vi "VI Messdaten-Verteiler.vi"(8 "error in (no error)":errorcluster caption="Fehler (Eingang, kein Fehler)") -> (0 "error out":errorcluster caption="Fehler (Ausgang)")   [LabVIEW 2020, in "Messdaten.lvlib"]
uses:
  Messdaten/Messdaten.lvlib
  Messdaten/Aktionen FGV Messdaten logging.ctl
  Seiten/Log Konfig/Aktionen Logdatei erstellen.ctl
  Seiten/FT-IR/FGV FT-IR Aktionen.ctl
  Allgemein/Zykluszeiterfassung Aktionen.ctl
  Seiten/System Einstellungen V2/Aktioen FGV System.ctl
  Messdaten/Aktionen FGV Messwerte zusammenfassen.ctl
  Seiten/FT-IR/FGV FT-IR Diagnose Aktionen.ctl
  Seiten/FT-IR/FGV FT-IR Gasliste Aktionen.ctl
  Status Analysatoren/Aktion Status Analysatoren.ctl
  Seiten/Log Konfig/Aktionen LogFile schreiben.ctl
  Seiten/Log Konfig/Aktionen Trigger.ctl
  Seiten/EL3000/Allgemeine VI/Aktion FGV Werte Standardanalysator.ctl
  Seiten/FT-IR/Algebraic Modul/FGV Algebraic Aktionen.ctl
  Seiten/FT-IR/Aktionen EVID-Codes.ctl
  Messdaten/Aktionen FGV Messdaten.ctl
  Seiten/Log Konfig/Log Sequence FGV Aktion.ctl
  Seiten/FT-IR/FT-IR.lvlib
  Seiten/FT-IR/TOOLweb Interface Library/TOOLweb Interface.lvlib
  cRIO/PC/Kommunikation mit cRIO.lvlib
  Seiten/Log Konfig/LogKonfig.lvlib
  Seiten/FT-IR/AK interface/AK-Interface.lvlib
  Allgemein/allgemeine Sub-VIs.lvlib
  Seiten/EL3000/PMA/PMA.lvlib
  Seiten/EL3000/FID/FID.lvlib
  Seiten/EL3000/Allgemeine VI/Allgemeine VI.lvlib
  Seiten/FT-IR/Algebraic Modul/Algebraic Modul.lvlib
  Seiten/Lambdasonde/Lambda_ Komm.lvlib
  Status Analysatoren/Status Analysatoren.lvlib
  Linearisierung V2/Linearisierung v2.lvlib
  <vilib>/Platform/TimedLoop/XDataNode/XDataNode.xnode
  <vilib>/Platform/TimedLoop/XDataNode/nitl_modes.ctl
  <vilib>/Platform/TimedLoop/XDataNode/XDNodeRunTimeDep.lvlib
  <vilib>/Platform/TimedLoop/XDataNode/wakeup.ctl
  <vilib>/Platform/TimedLoop/XDataNode/timing_clust.ctl
  Seiten/FT-IR/TOOLweb Interface Library/TOOLweb Interface Hilfs-VIs.lvlib
  Seiten/System Einstellungen V2/System Einstellungen V2.lvlib
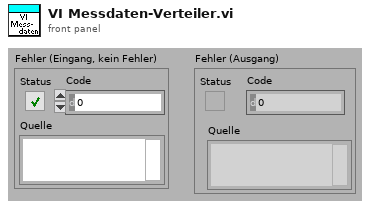
[diagram p1: front panel]
types:
  T1 = typedef "Messdaten.lvlib/Aktionen FGV Messdaten logging.ctl" = enum16{"lesen", "schreiben", "init", "löschen", "werte eintakten", "Flag setzen"}
  T2 = typedef "XDNodeRunTimeDep.lvlib/timing_clust.ctl" = cluster{"Expected End [f-1]":u64, "Actual End [f-1]":u64, "Finished Late? [f-1]":bool, "Expected End [i-1]":u64, "Actual End [i-1]":u64, "Finished Late? [i-1]":bool, "Expected Start [i]":u64, "Actual Start [i]":u64, "Expected Start [f]":u64, "Actual Start [f]":u64, "Source Name":string, "Structure Name":string, "Period":i64, "Deadline":i64, "Offset":i64, "Start":i64, "Priority":i32, "Timeout":i32, "Mode":T3, "Wakeup Reason":T4, "Error":errorcluster, "Source Type":string, "Secondary Source Type":string, "Global End Time":u64, "Global Start Time":u64, "Frame Duration":u64, "Iteration Duration":u64, "Assigned CPU":i32, "I/O Scan Engine Mode":u32}
  T3 = typedef "XDNodeRunTimeDep.lvlib/nitl_modes.ctl" = enum32{"No Change", "Process missed periods, maintain original phase", "Discard missed periods, maintain original phase", "Process missed periods, ignore original phase", "Discard missed periods, ignore original phase"}
  T4 = typedef "XDNodeRunTimeDep.lvlib/wakeup.ctl" = enum32{"Normal", "Aborted", "Asynchronous wakeup", "Timing source error", "Timed loop error", "Timeout"}
  T5 = typedef "System Einstellungen V2.lvlib/Aktioen FGV System.ctl" = enum16{"lesen", "laden", "speichern", "Optionen schreiben", "Zeitstempel", "Reset BMP", "Reset SQP", "Wartung", "Werkseinstellung"}
  T6 = typedef "allgemeine Sub-VIs.lvlib/Zykluszeiterfassung Aktionen.ctl" = enum16{"lesen", "init", "Messdaten1", "ToolWeb", "AK FT-IR", "AK Extern", "AK Amium"}
  T7 = typedef "FT-IR.lvlib/FGV FT-IR Aktionen.ctl" = enum16{"lesen", "NOG setzen", "NOS setzen", "Initialisieren", "speichern", "ALLES setzen", "FT-IR Spektrum loggen", "Komm Stoppen", "Spektrum LogKonfig"}
  T8 = typedef "Messdaten.lvlib/Aktionen FGV Messdaten.ctl" = enum16{"lesen", "schreiben", "löschen", "Mittelwerte", "Komponente"}
  T9 = typedef "FT-IR.lvlib/Aktionen EVID-Codes.ctl" = enum16{"lesen", "setzen", "laden", "speichern", "1Hz/5Hz", "Smoothing", "Rolling Average"}
  T10 = typedef "FT-IR.lvlib/Algebraic Modul.lvlib/FGV Algebraic Aktionen.ctl" = enum16{"lesen", "laden", "speichern", "berechnen", "schreiben"}
  T11 = typedef "ABB-EL3000.lvlib/Allgemeine VI.lvlib/Aktion FGV Werte Standardanalysator.ctl" = enum16{"lesen", "FID", "PMA"}
  T12 = typedef "Messdaten.lvlib/Aktionen FGV Messwerte zusammenfassen.ctl" = enum16{"lesen", "FT-IR", "Algebraic", "LabBaseName", "LabBaseNr"}
  T13 = typedef "LogKonfig.lvlib/Aktionen Trigger.ctl" = enum16{"lesen", "ALLE schreiben", "Trigger prüfen", "Trigger rücksetzen"}
  T14 = typedef "LogKonfig.lvlib/Log Sequence FGV Aktion.ctl" = enum16{"initialisieren", "lesen", "schreiben", "laden", "speichern", "übertragen"}
  T15 = typedef "FT-IR.lvlib/FGV FT-IR Gasliste Aktionen.ctl" = enum16{"lesen", "Gasliste FT-IR", "Gasliste ausgelesen", "laden", "speichern", "löschen"}
  T16 = typedef "System Einstellungen V2.lvlib/Optionen.ctl" = cluster{"Störmeldep.":bool, "Betriebszustände":bool, "AK in ppm":bool, "log Cal-Gas":bool, "log 0-Gas":bool, "Durchflusssensor 0-5V":bool, "PNS?":bool, "Mit N2 spülen":bool, "TRE08":bool, "Amium 10-Fach":bool, "Verticale Scrollbar aktiv":bool, "Loggingtakt":bool, "AK Rezeptwechsel gleich wie MKS":bool, "NG ECO":bool}
  T17 = typedef "Verwaltung - cRIO.lvlib/TC Eingaenge.ctl" = cluster{"TC0: Reserve":sgl, "TC1: HL zu FT-IR":sgl, "TC2: HL Extern SP1":sgl, "TC3: HL Extern SP2":sgl, "TC4: Reserve":sgl, "TC5: Reserve":sgl, "TC6: Reserve":sgl, "TC7: Reserve":sgl, "TC8: FT-IR":sgl, "TC9: Reserve":sgl, "TC10: Schaltschrank":sgl, "TC11: Umgebung":sgl}
  T18 = typedef "FT-IR.lvlib/Rolling Average Settings.ctl" = cluster{"Average":u32, "Average via AK:":bool, "Average IAG Software:":bool}
  T19 = typedef "Messdaten.lvlib/Rolling Average Daten.ctl" = cluster{"RA aktuelle Messwerte":sgl[], "RA Messdaten":sgl[][], "RA Deviation":sgl[], "RA Zeitstempeln":timestamp[], "Rohwerte FTIR":sgl[][]}
  T20 = typedef "String - Ausgabefeld.ctl" = string
  T21 = cluster{"Index Array":i32[], "Namen Array":string[], "Spektrum File Name":bool}
  T22 = typedef "LogKonfig.lvlib/Aktionen Logdatei erstellen.ctl" = enum16{"lesen", "Logdatei erstellen NEU", "Name NEU", "Pfad NEU", "Log Stop", "max Size"}
  T23 = typedef "LogKonfig.lvlib/Aktionen LogFile schreiben.ctl" = enum16{"lesen", "schreiben", "initialisieren"}
  T24 = typedef "LogKonfig.lvlib/Auswahlfeld aktiviert-deaktiviert.ctl" = u16
  T25 = typedef "Verwaltung - cRIO.lvlib/Digital Eingaenge 0-15.ctl" = cluster{"I0: N2 Nachf. FT-IR voll":bool, "I1: N2 Nachf. Vorrat leer":bool, "I2: (Klimaanlage eingeschaltet)":bool, "I3: (Klimaanlage Störung)":bool, "I4: Trigger Eingang (Messdaten sp.)":bool, "I5: Reserve":bool, "I6: Reserve":bool, "I7: Reserve":bool, "I8: Druckschalter Versorgung ok":bool, "I9: Reserve":bool, "I10: Reserve":bool, "I11: Reserve":bool, "I12: Drucksch. N2 Versorgung":bool, "I13: Reserve":bool, "I14: Drucksch. N2 Optikbox":bool, "I15: (Füllstand Kondensatbehälter)":bool}
  T26 = typedef "Status Analysatoren.lvlib/Aktion Status Analysatoren.ctl" = enum16{"lesen", "initialisieren", "Analysatoren aktiv", "FTIR Fehler", "FID Fehler", "PMA Fehler", "Felder einfärben"}
  T27 = typedef "FT-IR.lvlib/FGV FT-IR Diagnose Aktionen.ctl" = enum16{"Lesen", "Diagnose Schreiben", "Min Schreiben", "Max Schreiben"}
  T28 = typedef "FT-IR.lvlib/TOOLweb Interface.lvlib/Typdefinitionen.lvlib/TOOLweb Diagnose.ctl" = cluster{"(14) temperature":sgl, "(15) pressure":sgl, "(16) oxygen":sgl, "(50) diag-igramdc":sgl, "(51) diag-igrampp":sgl, "(52) diag-phaseAngle":sgl, "(53) diag-laserpp":sgl, "(54) diag-laserdc":sgl, "(55) diag-badscan":sgl, "(56) diag-centerburst":sgl, "(57) diag-linearizerCheck":sgl, "(58) diag-SNR":sgl, "(59) diag-sBeamIntensity":sgl}
  T29 = typedef "FT-IR.lvlib/TOOLweb Interface.lvlib/Typdefinitionen.lvlib/TOOLweb Einstellungen.ctl" = cluster{"(1) InstrumentState":string, "(10) NrOfGasses":i32, "(21) recipeCurrent":string, "(80) labEnabled":bool, "(81) labPath":path, "(82) labBaseName":string, "(83) labIndex":string, "(90) ftirScans":i32}
  T30 = cluster{"(80) labEnabled":bool, "(81) labPath":path, "(82) labBaseName":string, "(83) labIndex":string, "Spektrum loggen aktiv?":bool}
  T31 = typedef "Status Analysatoren.lvlib/Status.ctl" = cluster{"FT-IR aktiv":bool, "FT-IR Fehler":bool, "FID aktiv":bool, "FID Fehler":bool, "PMA aktiv":bool, "PMA Fehler":bool}
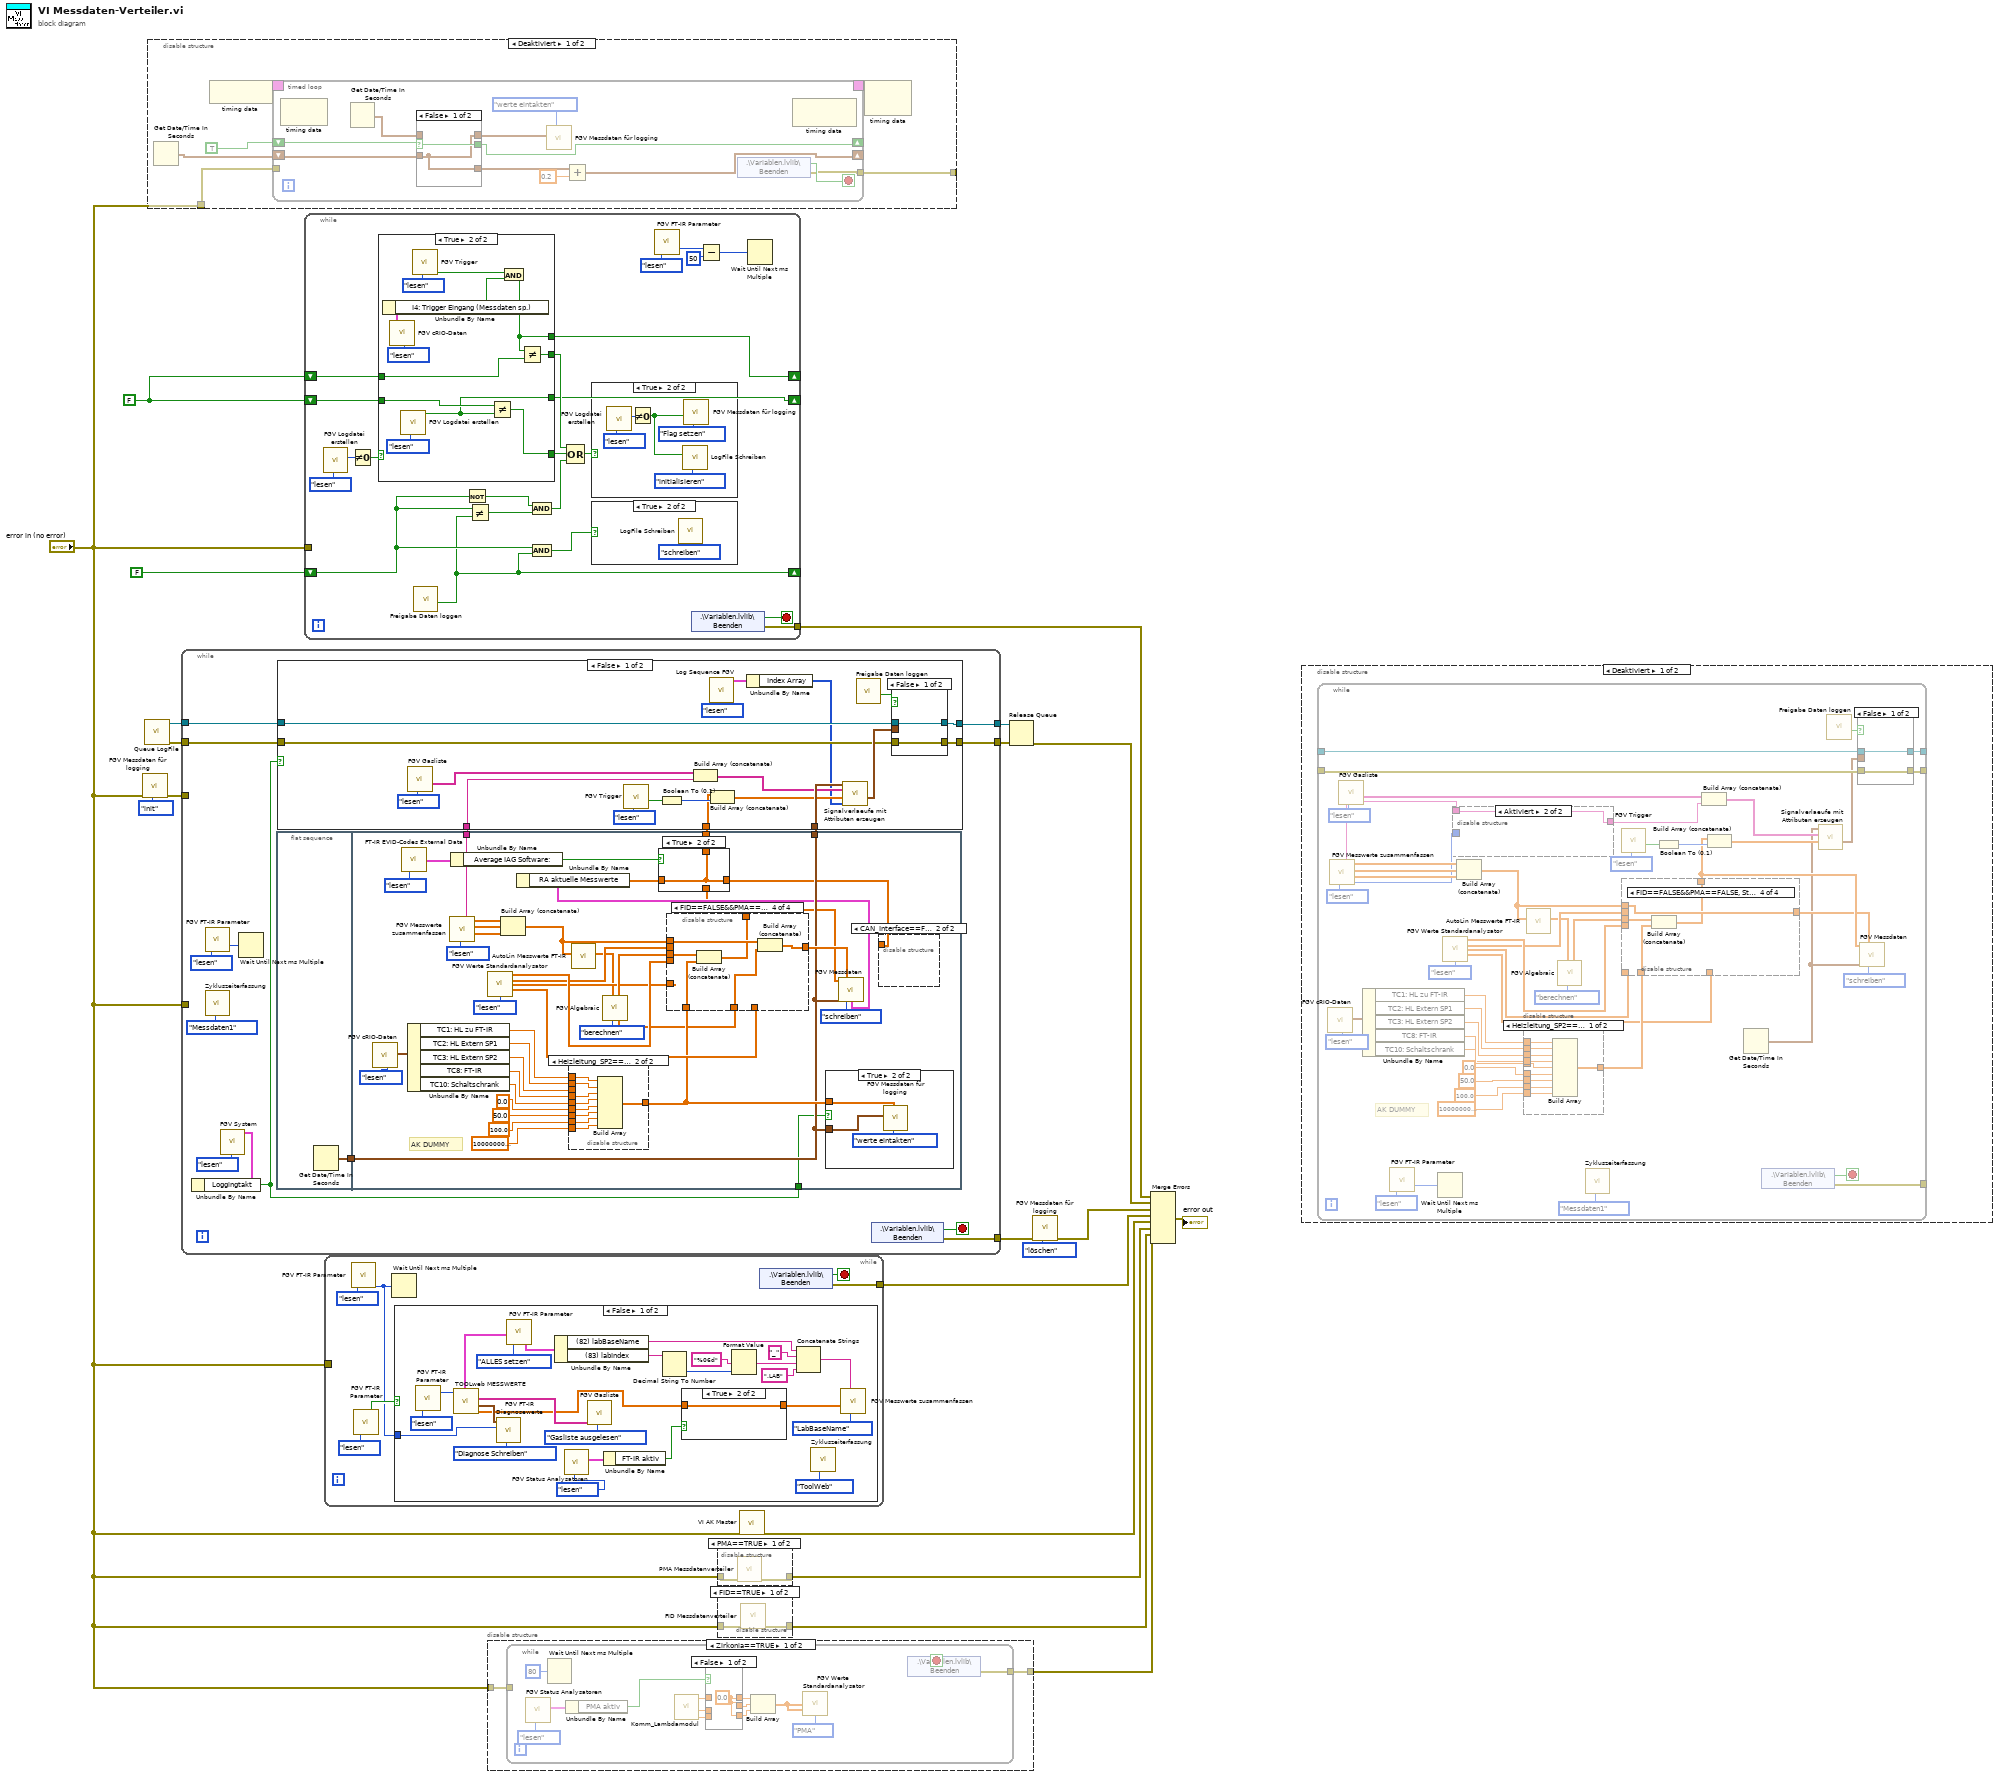
[diagram p0: block diagram]
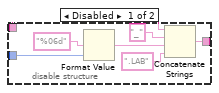
[diagram p2: hidden frame]
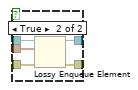
[diagram p3: hidden frame]
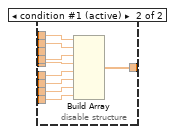
[diagram p4: hidden frame]
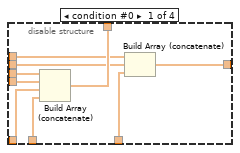
[diagram p5: hidden frame]
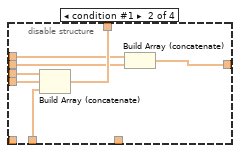
[diagram p6: hidden frame]
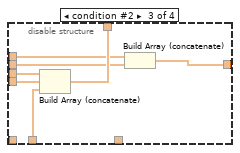
[diagram p7: hidden frame]
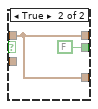
[diagram p9: hidden frame]
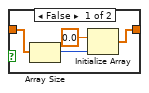
[diagram p13: hidden frame]
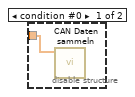
[diagram p20: hidden frame]
diagram:
  w12 = FALSE ("Daten loggen")
  n1 = call "FGV Messdaten für logging.vi"("Aktionen"=Aktionen_FGV_Messdaten_logging."init", "error in (no error)"="error in (no error)") -> ("error out"=w8:errorcluster)  [unwired: 9 in]
  n2 = call "Queue LogFile.vi"() -> ("error out"=w20:errorcluster, "Queue (Ausgang)"=w5:refnum<queue>)  [unwired: 6 in]
  n3 = disable-structure shown="Deaktiviert" {
    disable-tunnel: "error in (no error)" -> [w24 _]
    disable-tunnel: [w23 _] -> _
    frame Disabled {
      n4 = Get Date/Time In Seconds() -> (seconds since 1Jan1904=w22:timestamp)
      n5 = node-c288() -> (w26:T2)
      n6 = timed-loop {
        timing: w26 -> [_]
        timing-out: [_] -> w25
        tunnel: w24 -> [_]
        tunnel: [w36] -> w23
        shift-right: [w34] -> _
        shift-left: w22 -> [w32]
        shift-right: [w28] -> _
        shift-left: TRUE -> [w30]
        stop <- w37 stop-if-true
        n7 = node-c288() -> ()  [unwired: 1 in, 1 out]
        n8 = Get Date/Time In Seconds() -> (seconds since 1Jan1904=w29:timestamp)
        n9 = case shown="False" w30 {
          selector: w30 -> [w39 _]
          tunnel: w32 -> [w38 _]
          tunnel: [w38 w41] -> w31
          tunnel: w29 -> [_ w41]
          tunnel: [w38 w41] -> w27
          tunnel: [w39 FALSE] -> w28
          frame False {
          }
          frame True {
          }
        }
        n10 = call "FGV Messdaten für logging.vi"("Temp/Konst."=Aktionen_FGV_Messdaten_logging."werte eintakten" ("Aktionen"), "Aktuelle Zeit"=w27) -> ()  [unwired: 9 in, 1 out]
        n11 = Add(x=w31, y=0.2) -> (x+y=w34:timestamp)
        n12 = shared-variable ".\\Variablen.lvlib\\Beenden"() -> (w37:bool, error out=w36:errorcluster)  [unwired: 1 out]
        n13 = node-c288() -> ()  [unwired: 1 in, 1 out]
      }
      n14 = node-c288(w25) -> ()  [unwired: 1 out]
    }
    frame Enabled {
    }
  }
  n15 = while {
    tunnel: w20 -> [w51]
    tunnel: [w58] -> w11
    tunnel: "error in (no error)" -> [_]
    tunnel: w8 -> [_]
    tunnel: w5 -> [w52]
    tunnel: [w50] -> w4
    tunnel: [w49] -> w3
    stop <- w61 stop-if-true
    n16 = call "FGV FT-IR Parameter.vi"("Aktion"=FGV_FT-IR_Aktionen."lesen") -> ("Zykluszeit Messdatenverteiler"=w59:u32)  [unwired: 11 in, 7 out]
    n17 = call "Zykluszeiterfassung.vi"("Aktionen"=Zykluszeiterfassung_Aktionen."Messdaten1") -> ()  [unwired: 10 in, 1 out]
    n18 = call "FGV System.vi"("Aktionen"=Aktioen_FGV_System."lesen") -> ("Optionen"=w56:T16)  [unwired: 12 in, 6 out]
    n19 = Unbundle By Name(w56) -> ("Loggingtakt"=w46:bool)
    n20 = Wait Until Next ms Multiple(millisecond multiple=w59) -> ()  [unwired: 1 out]
    n21 = flat-sequence {
      tunnel: [w62] -> w48
      tunnel: [w101] -> w54
      tunnel: [w68] -> w53
      tunnel: w48 -> [w74]
      tunnel: [w74] -> w47
      tunnel: w46 -> [w73]
      frame #0 {
        n22 = Get Date/Time In Seconds() -> (seconds since 1Jan1904=w62:timestamp)
      }
      frame #1 {
        # "AK DUMMY"
        n23 = call "FGV cRIO-Daten.vi"("Aktion"=enum16{"lesen", "schreiben"}."lesen") -> ("TC Eingänge"=w84:T17)  [unwired: 9 in, 9 out]
        n24 = call "FT-IR EVID-Codes External Data.vi"("Aktionen"=Aktionen_EVID-Codes."lesen") -> ("Rolling Average Settings"=w66:T18)  [unwired: 9 in, 5 out]
        n25 = Unbundle By Name(w84) -> ("TC1: HL zu FT-IR"=w99:sgl, "TC2: HL Extern SP1"=w98:sgl, "TC3: HL Extern SP2"=w97:sgl, "TC8: FT-IR"=w77:sgl, "TC10: Schaltschrank"=w96:sgl)
        n26 = call "FGV Messwerte zusammenfassen.vi"("Aktionen"=Aktionen_FGV_Messwerte_zusammenfassen."lesen") -> ("FTIR Status"=w88:sgl[], "Algebraic"=w89:sgl[], "FT-IR"=w76:sgl[], "labBaseName"=w101:string)  [unwired: 6 in, 1 out]
        n27 = Unbundle By Name(w66) -> ("Average IAG Software:"=w65:bool)
        n28 = call "FGV Werte Standardanalysator.vi"("Aktion"=Aktion_FGV_Werte_Standardanalysator."lesen") -> ("FID"=w83:sgl[], "FID Rohwerte"=w82:sgl[], "PMA"=w81:sgl[], "PMA Rohwerte"=w80:sgl[])  [unwired: 8 in, 3 out]
        n29 = Build Array (concatenate)(w76, w89, w88) -> (w86:sgl[])
        n30 = disable-structure shown="Heizleitung_SP2==FALSE, Standard" {
          disable-tunnel: w99 -> [w117 w126]
          disable-tunnel: w98 -> [w116 w125]
          disable-tunnel: w97 -> [w115 _]
          disable-tunnel: w96 -> [w114 w124]
          disable-tunnel: sgl 0.0 ("Element") -> [w113 w123]
          disable-tunnel: sgl 100.0 ("Element") -> [w112 w122]
          disable-tunnel: sgl 10000000000.0 ("Element") -> [w111 w121]
          disable-tunnel: sgl 50.0 ("Element") -> [w110 w120]
          disable-tunnel: [w109 w119] -> w75
          disable-tunnel: w77 -> [w108 w118]
          frame condition #0 {
            n31 = Build Array(w117, w116, w115, w108, w114, w113, w110, w112, w111) -> (w109:sgl[])
          }
          frame condition #1 (active) {
            n32 = Build Array(w126, w125, w118, w124, w123, w120, w122, w121) -> (w119:sgl[])
          }
        }
        n33 = call "AutoLin Messwerte FT-IR.vi"("FT-IR Rohwerte"=w86) -> ("FT-IR Linearisiert"=w79:sgl[])  [unwired: 10 in]
        n34 = call "FGV Algebraic.vi"("Aktionen Algebraic"=FGV_Algebraic_Aktionen."berechnen", "Istwerte"=w79) -> ("Rohwerte"=w72:sgl[], "Messdaten"=w90:sgl[])  [unwired: 5 in, 3 out]
        n35 = disable-structure shown="FID==FALSE&&PMA==FALSE, Standard" {
          disable-tunnel: [w135 w142 w149 w153] -> w69
          disable-tunnel: w90 -> [w134 w141 w148 w155]
          disable-tunnel: w75 -> [w133 w140 w147 w152]
          disable-tunnel: w86 -> [w132 w139 w146 w154]
          disable-tunnel: [w131 w138 w145 w151] -> w85
          disable-tunnel: w83 -> [w130 _ w144 _]
          disable-tunnel: w82 -> [w129 _ w143 _]
          disable-tunnel: w81 -> [w128 w136 _ _]
          disable-tunnel: w80 -> [w127 w137 _ _]
          disable-tunnel: w72 -> [_ _ _ w150]
          frame condition #0 {
            n36 = Build Array (concatenate)(w134, w130, w128, w133) -> (w135:sgl[])
            n37 = Build Array (concatenate)(w132, w129, w127) -> (w131:sgl[])
          }
          frame condition #1 {
            n38 = Build Array (concatenate)(w141, w136, w140) -> (w142:sgl[])
            n39 = Build Array (concatenate)(w139, w137) -> (w138:sgl[])
          }
          frame condition #2 {
            n40 = Build Array (concatenate)(w148, w144, w147) -> (w149:sgl[])
            n41 = Build Array (concatenate)(w146, w143) -> (w145:sgl[])
          }
          frame condition #3 (active) {
            n42 = Build Array (concatenate)(w155, w152) -> (w153:sgl[])
            n43 = Build Array (concatenate)(w154, w150) -> (w151:sgl[])
          }
        }
        n44 = case shown="True" w73 {
          tunnel: w74 -> [_ w106]
          tunnel: w75 -> [_ w105]
          frame False {
          }
          frame True {
            n45 = call "FGV Messdaten für logging.vi"("Aktionen"=Aktionen_FGV_Messdaten_logging."werte eintakten", "Temp/Konst."=w105, "Aktuelle Zeit"=w106) -> ()  [unwired: 8 in, 1 out]
          }
        }
        n46 = call "FGV Messdaten.vi"("Neue Messwerte"=w69, "Rohwerte"=w85, "Neuer Zeitstempel"=w74, "Aktionen"=Aktionen_FGV_Messdaten."schreiben") -> ("Ausgangs-Cluster"=w71:T19)  [unwired: 3 in, 8 out]
        n47 = Unbundle By Name(w71) -> ("RA aktuelle Messwerte"=w70:sgl[])
        n48 = case shown="True" w65 {
          tunnel: w70 -> [_ w104]
          tunnel: w69 -> [w103 _]
          tunnel: [w103 w104] -> w68
          tunnel: [w103 w104] -> w63
          frame False {
          }
          frame True {
          }
        }
        n49 = disable-structure shown="CAN_Interface==FALSE" {
          disable-tunnel: w63 -> [w102 _]
          frame condition #0 {
            n50 = call "CAN Daten sammeln.vi"("Aktuelle Messwerte"=w102) -> ()  [unwired: 11 in]
          }
          frame condition #1 (active) {
          }
        }
      }
    }
    n51 = case shown="False" w46 {
      tunnel: w54 -> [w160 _]
      tunnel: w53 -> [w170 _]
      tunnel: w47 -> [w169 _]
      tunnel: w52 -> [w164 _]
      tunnel: w51 -> [w163 _]
      tunnel: [w162 _] -> w50
      tunnel: [w161 _] -> w49
      frame False {
        n52 = call "FGV Gasliste.vi"("Aktionen"=FGV_FT-IR_Gasliste_Aktionen."lesen") -> ("Aktuelle Gasliste gesamt"=w173:T20[])  [unwired: 8 in, 2 out]
        n53 = call "FGV Trigger.vi"("Aktion"=Aktionen_Trigger."lesen") -> ("Trigger gesetzt?"=w172:bool)  [unwired: 7 in, 3 out]
        n54 = Boolean To (0,1)(Boolean=w172) -> (0, 1=w171:i16)
        n55 = Build Array (concatenate)(w173, w160) -> (w168:T20[])
        n56 = call "Log Sequence FGV.vi"("Aktion"=Log_Sequence_FGV_Aktion."lesen") -> ("Cluster (out)"=w159:T21)  [unwired: 10 in]
        n57 = Build Array (concatenate)(w170, w171) -> (w167:sgl[])
        n58 = Unbundle By Name(w159) -> ("Index Array"=w158:i32[])
        n59 = call "Signalverlaeufe mit Attributen erzeugen.vi"("Log Sequence"=w158, "Messwerte"=w167, "Namen"=w168, "Zeitstempel"=w169) -> ("Signalverläufe"=w165:waveform(dbl)[])  [unwired: 7 in]
        n60 = call "Freigabe Daten loggen.vi"() -> ("Daten loggen"=w166:bool)  [unwired: 11 in]
        n61 = case shown="False" w166 {
          tunnel: w164 -> [w176 w181]
          tunnel: [w176 w180] -> w162
          tunnel: [w175 w179] -> w161
          tunnel: w163 -> [w175 w178]
          tunnel: w165 -> [_ w177]
          frame False {
          }
          frame True {
            n62 = Lossy Enqueue Element(queue=w181, element=w177, error in (no error)=w178) -> (queue out=w180:refnum<queue>, error out=w179:errorcluster)  [unwired: 2 out]
          }
        }
      }
      frame True {
      }
    }
    n63 = shared-variable ".\\Variablen.lvlib\\Beenden"() -> (w61:bool, error out=w58:errorcluster)  [unwired: 1 out]
  }
  n64 = while {
    shift-right: [w200] -> _
    shift-left: FALSE ("Daten loggen") -> [w201]
    tunnel: [w197] -> w2
    tunnel: "error in (no error)" -> [_]
    shift-right: [w186] -> _
    shift-left: w12 -> [w187]
    shift-right: [w189] -> _
    shift-left: w12 -> [w190]
    stop <- w198 stop-if-true
    n65 = call "FGV Logdatei erstellen.vi"("Aktion"=Aktionen_Logdatei_erstellen."lesen") -> ("Logdatei erstellen neu"=w183:T24)  [unwired: 6 in, 4 out]
    n66 = Not Equal To 0?(x=w183) -> (x != 0?=w182:bool)
    n67 = case shown="True" w182 {
      tunnel: w190 -> [_ w210]
      tunnel: [_ w209] -> w189
      tunnel: [_ w208] -> w188
      tunnel: w187 -> [_ w206]
      tunnel: [_ w205] -> w186
      tunnel: [_ w204] -> w185
      frame False {
      }
      frame True {
        n68 = call "FGV cRIO-Daten.vi"("Aktion"=enum16{"lesen", "schreiben"}."lesen") -> ("DI"=w212:T25)  [unwired: 9 in, 9 out]
        n69 = Unbundle By Name(w212) -> ("I4: Trigger Eingang (Messdaten sp.)"=w211:bool)
        n70 = call "FGV Logdatei erstellen.vi"("Aktion"=Aktionen_Logdatei_erstellen."lesen") -> ("Loggen stoppen"=w205:bool)  [unwired: 6 in, 4 out]
        n71 = call "FGV Trigger.vi"("Aktion"=Aktionen_Trigger."lesen") -> ("Trigger Eingang"=w214:bool)  [unwired: 7 in, 3 out]
        n72 = Not Equal?(x=w206, y=w205) -> (x != y?=w204:bool)
        n73 = And(x=w214, y=w211) -> (x .and. y?=w209:bool)
        n74 = Not Equal?(x=w209, y=w210) -> (x != y?=w208:bool)
      }
    }
    n75 = call "Freigabe Daten loggen.vi"() -> ("Daten loggen"=w200:bool)  [unwired: 11 in]
    n76 = Not(x=w201) -> (.not. x?=w203:bool)
    n77 = Not Equal?(x=w201, y=w200) -> (x != y?=w202:bool)
    n78 = And(x=w203, y=w202) -> (x .and. y?=w191:bool)
    n79 = And(x=w201, y=w200) -> (x .and. y?=w199:bool)
    n80 = Compound Arithmetic op=OR ("Mehrfacharithmetik")(w188, w185, w191) -> (w192:bool)
    n81 = case shown="True" w192 {
      frame False {
      }
      frame True {
        n82 = call "FGV Logdatei erstellen.vi"("Aktion"=Aktionen_Logdatei_erstellen."lesen") -> ("Logdatei erstellen neu"=w219:T24)  [unwired: 6 in, 4 out]
        n83 = Not Equal To 0?(x=w219) -> (x != 0?=w217:bool)
        n84 = call "LogFile Schreiben.vi"("Aktion"=Aktionen_LogFile_schreiben."initialisieren", "LogFile erstellen?"=w217) -> ()  [unwired: 6 in, 4 out]
        n85 = call "FGV Messdaten für logging.vi"("Aktionen"=Aktionen_FGV_Messdaten_logging."Flag setzen", "Boolesch"=w217) -> ()  [unwired: 9 in, 1 out]
      }
    }
    n86 = case shown="True" w199 {
      frame False {
      }
      frame True {
        n87 = call "LogFile Schreiben.vi"("Aktion"=Aktionen_LogFile_schreiben."schreiben") -> ()  [unwired: 7 in, 4 out]
      }
    }
    n88 = call "FGV FT-IR Parameter.vi"("Aktion"=FGV_FT-IR_Aktionen."lesen") -> ("Zykluszeit Messdatenverteiler"=w195:u32)  [unwired: 11 in, 7 out]
    n89 = shared-variable ".\\Variablen.lvlib\\Beenden"() -> (w198:bool, error out=w197:errorcluster)  [unwired: 1 out]
    n90 = Subtract(x=w195, y=u32 50) -> (x-y=w193:u32)
    n91 = Wait Until Next ms Multiple(millisecond multiple=w193) -> ()  [unwired: 1 out]
  }
  n92 = while {
    tunnel: [w226] -> w19
    tunnel: "error in (no error)" -> [_]
    stop <- w227 stop-if-true
    n93 = call "FGV FT-IR Parameter.vi"("Aktion"=FGV_FT-IR_Aktionen."lesen") -> ("Zykluszeit ToolWeb"=w222:u32)  [unwired: 11 in, 7 out]
    n94 = call "FGV FT-IR Parameter.vi"("Aktion"=FGV_FT-IR_Aktionen."lesen") -> ("Komm Stoppen"=w224:bool)  [unwired: 11 in, 7 out]
    n95 = Wait Until Next ms Multiple(millisecond multiple=w222) -> ()  [unwired: 1 out]
    n96 = case shown="False" w224 {
      tunnel: w222 -> [w236 _]
      frame False {
        n97 = call "FGV FT-IR Parameter.vi"("Aktion"=FGV_FT-IR_Aktionen."lesen") -> ("NoOfGasses"=w251:u32)  [unwired: 11 in, 7 out]
        n98 = call "TOOLweb MESSWERTE.vi"("Anzahl Gase"=w251) -> ("Status"=w240:sgl[], "Diagnose"=w248:T28, "gas#label"=w249:string[], "Einstellungen"=w244:T29)  [unwired: 6 in, 1 out]
        n99 = call "FGV FT-IR Diagnosewerte.vi"("Aktionen"=FGV_FT-IR_Diagnose_Aktionen."Diagnose Schreiben", "Zykluszeit ToolWeb"=w236, "Diagnose neu"=w248) -> ()  [unwired: 3 in, 6 out]
        n100 = call "FGV FT-IR Parameter.vi"("Einstellungen"=w244, "Aktion"=FGV_FT-IR_Aktionen."ALLES setzen") -> ("Ausgangs-Cluster"=w243:T30)  [unwired: 10 in, 7 out]
        n101 = Unbundle By Name(w243) -> ("(82) labBaseName"=w230:string, "(83) labIndex"=w232:string)
        n102 = call "FGV Status Analysatoren.vi"("Aktionen"=Aktion_Status_Analysatoren."lesen") -> ("Status Analysatoren"=w239:T31)  [unwired: 10 in]
        n103 = call "FGV Gasliste.vi"("Aktionen"=FGV_FT-IR_Gasliste_Aktionen."Gasliste ausgelesen", "Gasliste ausgelesen"=w249) -> ()  [unwired: 7 in, 3 out]
        n104 = Unbundle By Name(w239) -> ("FT-IR aktiv"=w237:bool)
        n105 = Decimal String To Number(string=w232) -> (number=w231:i32)  [unwired: 2 in, 1 out]
        n106 = case shown="True" w237 {
          tunnel: w240 -> [w256 w257]
          tunnel: [w253 w257] -> w241
          frame False {
            n107 = Array Size(array=w256) -> (size(s)=w255:i32)
            n108 = Initialize Array(sgl 0.0 ("Element"), w255) -> (w253:sgl[])
          }
          frame True {
          }
        }
        n109 = Format Value(format string="%06d" ("Format-String"), value (0)=w231) -> (output string=w234:string)  [unwired: 1 in]
        n110 = Concatenate Strings(w230, "_" ("String"), w234, ".LAB" ("String")) -> (w229:string)
        n111 = call "Zykluszeiterfassung.vi"("Aktionen"=Zykluszeiterfassung_Aktionen."ToolWeb") -> ()  [unwired: 10 in, 1 out]
        n112 = call "FGV Messwerte zusammenfassen.vi"("Aktionen"=Aktionen_FGV_Messwerte_zusammenfassen."LabBaseName", "labBaseName"=w229, "FTIR Status"=w241) -> ()  [unwired: 4 in, 5 out]
      }
      frame True {
      }
    }
    n113 = shared-variable ".\\Variablen.lvlib\\Beenden"() -> (w227:bool, error out=w226:errorcluster)  [unwired: 1 out]
  }
  n114 = disable-structure shown="Zirkonia==TRUE" {
    disable-tunnel: [w259 _] -> w13
    disable-tunnel: "error in (no error)" -> [w258 _]
    frame condition #0 {
      n115 = while {
        tunnel: [w272] -> w259
        tunnel: w258 -> [_]
        stop <- w273 stop-if-true
        n116 = call "FGV Status Analysatoren.vi"("Aktionen"=Aktion_Status_Analysatoren."lesen") -> ("Status Analysatoren"=w268:T31)  [unwired: 10 in]
        n117 = Wait Until Next ms Multiple(millisecond multiple=u32 80 ("ms")) -> ()  [unwired: 1 out]
        n118 = Unbundle By Name(w268) -> ("PMA aktiv"=w260:bool)
        n119 = call "Komm_Lambdamodul.vi"() -> ("A/F"=w262:sgl, "O2"=w264:sgl, "Lambda"=w265:sgl)  [unwired: 8 in, 1 out]
        n120 = case shown="False" w260 {
          tunnel: [w274 w277] -> w266
          tunnel: w265 -> [_ w277]
          tunnel: w264 -> [_ w276]
          tunnel: [w274 w276] -> w263
          tunnel: w262 -> [_ w275]
          tunnel: [w274 w275] -> w261
          frame False {
            w274 = sgl 0.0 ("Lambda")
          }
          frame True {
          }
        }
        n121 = Build Array(w266, w263, w261) -> (w270:sgl[])
        n122 = call "FGV Werte Standardanalysator.vi"("PMA"=w270, "PMA Rohwerte"=w270, "Aktion"=Aktion_FGV_Werte_Standardanalysator."PMA") -> ()  [unwired: 6 in, 7 out]
        n123 = shared-variable ".\\Variablen.lvlib\\Beenden"() -> (w273:bool, error out=w272:errorcluster)  [unwired: 1 out]
      }
    }
    frame condition #1 (active) {
    }
  }
  n124 = disable-structure shown="PMA==TRUE" {
    disable-tunnel: [w279 _] -> w15
    disable-tunnel: "error in (no error)" -> [w278 _]
    frame condition #0 {
      n125 = call "PMA Messdatenverteiler.vi"("error IO"=w278) -> ("error IO"=w279:errorcluster)  [unwired: 10 in]
    }
    frame condition #1 (active) {
    }
  }
  n126 = disable-structure shown="FID==TRUE" {
    disable-tunnel: [w281 _] -> w14
    disable-tunnel: "error in (no error)" -> [w280 _]
    frame condition #0 {
      n127 = call "FID Messdatenverteiler.vi"("error in (no error)"=w280) -> ("error out"=w281:errorcluster)  [unwired: 10 in]
    }
    frame condition #1 (active) {
    }
  }
  n128 = call "VI AK Master.vi"("error in (no error)"="error in (no error)") -> ("error out"=w16:errorcluster)  [unwired: 10 in]
  n129 = Release Queue(queue=w4, error in (no error)=w3) -> (error out=w1:errorcluster)  [unwired: 3 out]
  n130 = call "FGV Messdaten für logging.vi"("Aktionen"=Aktionen_FGV_Messdaten_logging."löschen", "error in (no error)"=w11) -> ("error out"=w10:errorcluster)  [unwired: 9 in]
  n131 = Merge Errors(w2, w1, w10, w19, w16, w15, w14, w13) -> (→"error out":errorcluster)
  n132 = disable-structure shown="Deaktiviert" {
    frame Disabled {
      n133 = while {
        tunnel: _ -> [w331]
        tunnel: _ -> [w329]
        tunnel: [w330] -> _
        tunnel: [w328] -> _
        tunnel: [w308] -> _
        stop <- w327 stop-if-true
        # "AK DUMMY"
        n134 = call "FGV cRIO-Daten.vi"("Aktion"=enum16{"lesen", "schreiben"}."lesen") -> ("TC Eingänge"=w297:T17)  [unwired: 9 in, 9 out]
        n135 = call "FGV Messwerte zusammenfassen.vi"("Aktionen"=Aktionen_FGV_Messwerte_zusammenfassen."lesen") -> ("LabBaseNr"=w284:i32, "FTIR Status"=w302:sgl[], "Algebraic"=w303:sgl[], "FT-IR"=w285:sgl[], "labBaseName"=w292:string)  [unwired: 6 in]
        n136 = call "FGV Gasliste.vi"("Aktionen"=FGV_FT-IR_Gasliste_Aktionen."lesen") -> ("Aktuelle Gasliste gesamt"=w315:T20[])  [unwired: 8 in, 2 out]
        n137 = Unbundle By Name(w297) -> ("TC1: HL zu FT-IR"=w325:sgl, "TC2: HL Extern SP1"=w324:sgl, "TC3: HL Extern SP2"=w323:sgl, "TC8: FT-IR"=w287:sgl, "TC10: Schaltschrank"=w322:sgl)
        n138 = call "FGV FT-IR Parameter.vi"("Aktion"=FGV_FT-IR_Aktionen."lesen") -> ("Zykluszeit Messdatenverteiler"=w310:u32)  [unwired: 11 in, 7 out]
        n139 = Wait Until Next ms Multiple(millisecond multiple=w310) -> ()  [unwired: 1 out]
        n140 = call "FGV Werte Standardanalysator.vi"("Aktion"=Aktion_FGV_Werte_Standardanalysator."lesen") -> ("FID"=w296:sgl[], "FID Rohwerte"=w295:sgl[], "PMA"=w294:sgl[], "PMA Rohwerte"=w293:sgl[])  [unwired: 8 in, 3 out]
        n141 = disable-structure shown="Aktiviert" {
          disable-tunnel: w292 -> [w338 w339]
          disable-tunnel: [w337 w339] -> w291
          disable-tunnel: w284 -> [w332 _]
          frame Disabled {
            n142 = Format Value(format string="%06d" ("Format-String"), value (0)=w332) -> (output string=w335:string)  [unwired: 1 in]
            n143 = Concatenate Strings(w338, "_" ("String"), w335, ".LAB" ("String")) -> (w337:string)
          }
          frame Enabled {
          }
        }
        n144 = Build Array (concatenate)(w285, w303, w302) -> (w299:sgl[])
        n145 = disable-structure shown="Heizleitung_SP2==TRUE" {
          disable-tunnel: w325 -> [w356 w365]
          disable-tunnel: w324 -> [w355 w364]
          disable-tunnel: w323 -> [w354 _]
          disable-tunnel: w322 -> [w353 w363]
          disable-tunnel: sgl 0.0 ("Element") -> [w352 w362]
          disable-tunnel: sgl 100.0 ("Element") -> [w351 w361]
          disable-tunnel: sgl 10000000000.0 ("Element") -> [w350 w360]
          disable-tunnel: sgl 50.0 ("Element") -> [w349 w359]
          disable-tunnel: [w348 w358] -> w304
          disable-tunnel: w287 -> [w347 w357]
          frame condition #0 {
            n146 = Build Array(w356, w355, w354, w347, w353, w352, w349, w351, w350) -> (w348:sgl[])
          }
          frame condition #1 (active) {
            n147 = Build Array(w365, w364, w357, w363, w362, w359, w361, w360) -> (w358:sgl[])
          }
        }
        n148 = call "AutoLin Messwerte FT-IR.vi"("FT-IR Rohwerte"=w299) -> ("FT-IR Linearisiert"=w289:sgl[])  [unwired: 10 in]
        n149 = call "FGV Algebraic.vi"("Aktionen Algebraic"=FGV_Algebraic_Aktionen."berechnen", "Istwerte"=w289) -> ("Messdaten"=w305:sgl[])  [unwired: 5 in, 4 out]
        n150 = call "Zykluszeiterfassung.vi"("Aktionen"=Zykluszeiterfassung_Aktionen."Messdaten1") -> ()  [unwired: 10 in, 1 out]
        n151 = call "FGV Trigger.vi"("Aktion"=Aktionen_Trigger."lesen") -> ("Trigger gesetzt?"=w312:bool)  [unwired: 7 in, 3 out]
        n152 = disable-structure shown="FID==FALSE&&PMA==FALSE, Standard" {
          disable-tunnel: [w374 w381 w388 w390] -> w306
          disable-tunnel: w305 -> [w373 w380 w387 w392]
          disable-tunnel: w304 -> [w372 w379 w386 w389]
          disable-tunnel: w299 -> [w371 w378 w385 w391]
          disable-tunnel: [w370 w377 w384 w391] -> w298
          disable-tunnel: w296 -> [w369 w376 w383 _]
          disable-tunnel: w295 -> [w368 w375 w382 _]
          disable-tunnel: w294 -> [w367 _ _ _]
          disable-tunnel: w293 -> [w366 _ _ _]
          frame condition #0 {
            n153 = Build Array (concatenate)(w373, w369, w367, w372) -> (w374:sgl[])
            n154 = Build Array (concatenate)(w371, w368, w366) -> (w370:sgl[])
          }
          frame condition #1 {
            n155 = Build Array (concatenate)(w380, w376, w379) -> (w381:sgl[])
            n156 = Build Array (concatenate)(w378, w375) -> (w377:sgl[])
          }
          frame condition #2 {
            n157 = Build Array (concatenate)(w387, w383, w386) -> (w388:sgl[])
            n158 = Build Array (concatenate)(w385, w382) -> (w384:sgl[])
          }
          frame condition #3 (active) {
            n159 = Build Array (concatenate)(w392, w389) -> (w390:sgl[])
          }
        }
        n160 = Boolean To (0,1)(Boolean=w312) -> (0, 1=w311:i16)
        n161 = Build Array (concatenate)(w315, w291) -> (w317:T20[])
        n162 = Build Array (concatenate)(w306, w311) -> (w316:sgl[])
        n163 = Get Date/Time In Seconds() -> (seconds since 1Jan1904=w286:timestamp)
        n164 = shared-variable ".\\Variablen.lvlib\\Beenden"() -> (w327:bool, error out=w308:errorcluster)  [unwired: 1 out]
        n165 = call "Signalverlaeufe mit Attributen erzeugen.vi"("Messwerte"=w316, "Namen"=w317, "Zeitstempel"=w286) -> ("Signalverläufe"=w283:waveform(dbl)[])  [unwired: 8 in]
        n166 = call "Freigabe Daten loggen.vi"() -> ("Daten loggen"=w282:bool)  [unwired: 11 in]
        n167 = case shown="False" w282 {
          tunnel: w331 -> [w341 w346]
          tunnel: [w341 w345] -> w330
          tunnel: [w340 w344] -> w328
          tunnel: w329 -> [w340 w343]
          tunnel: w283 -> [_ w342]
          frame False {
          }
          frame True {
            n168 = Lossy Enqueue Element(queue=w346, element=w342, error in (no error)=w343) -> (queue out=w345:refnum<queue>, error out=w344:errorcluster)  [unwired: 2 out]
          }
        }
        n169 = call "FGV Messdaten.vi"("Neue Messwerte"=w306, "Rohwerte"=w298, "Neuer Zeitstempel"=w286, "Aktionen"=Aktionen_FGV_Messdaten."schreiben") -> ()  [unwired: 3 in, 9 out]
      }
    }
    frame Enabled {
    }
  }
